vi "Process.vi"(4 "Normalize?":bool, 5 "Measurement Arrays IN":T1, 6 "Calibration Constant (1/deg)":dbl, 7 "Magnet position":dbl, 8 "Magnetic Field (mT)":dbl, 9 "Actual Measurement":T2={"Elapsed Time (s)"=0.0, "Hall sensor (mT)"=0.0, "LockIn A"=[1.33515e-05, 1.14442e-05, 1.90736e-05, 41.634], "LockIn B"=[1.33515e-05, 1.14442e-05, 1.90736e-05, 41.634], "Dc intensity (V)"=0.0, "Temperature (K)"=0.0}) -> (3 "Measurement Arrays OUT":T1)   [LabVIEW 2017]
uses:
  Meas_arrays.ctl
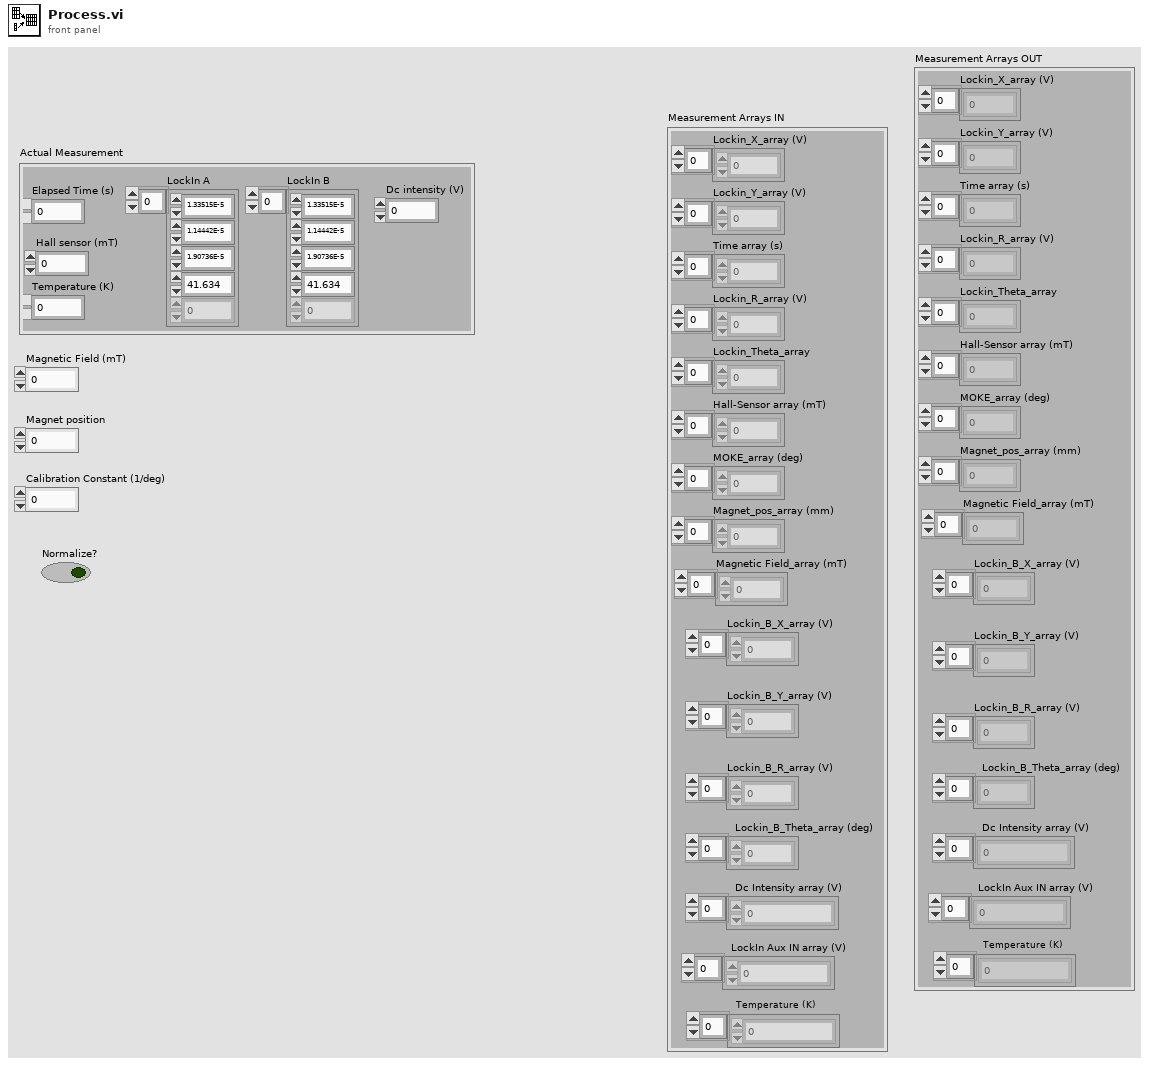
[diagram p1: front panel]
types:
  T1 = typedef "Meas_arrays.ctl" = cluster{"Lockin_X_array (V)":dbl[], "Lockin_Y_array (V)":dbl[], "Time array (s)":dbl[], "Lockin_R_array (V)":dbl[], "Lockin_Theta_array":dbl[], "Hall-Sensor array (mT)":dbl[], "MOKE_array (deg)":dbl[], "Magnet_pos_array (mm)":dbl[], "Magnetic Field_array (mT)":dbl[], "Lockin_B_X_array (V)":dbl[], "Lockin_B_Y_array (V)":dbl[], "Lockin_B_R_array (V)":dbl[], "Lockin_B_Theta_array (deg)":dbl[], "Dc Intensity array (V)":dbl[], "LockIn Aux IN array (V)":dbl[], "Temperature (K)":dbl[]}
  T2 = cluster{"Elapsed Time (s)":dbl, "Hall sensor (mT)":dbl, "LockIn A":dbl[], "LockIn B":dbl[], "Dc intensity (V)":dbl, "Temperature (K)":dbl}
  T3 = cluster{"Lockin_X_array (V)":dbl[], "Lockin_Y_array (V)":dbl[], "Time array (s)":dbl[], "Lockin_R_array (V)":dbl[], "Lockin_Theta_array":dbl[], "Hall-Sensor array (mT)":dbl[], "MOKE_array (deg)":dbl[], "Magnet_pos_array (mm)":dbl[], "Magnetic Field_array (mT)":dbl[], "Lockin_B_X_array (V)":dbl[], "Lockin_B_Y_array (V)":dbl[], "Lockin_B_R_array (V)":dbl[], "Lockin_B_Theta_array (deg)":dbl[], "Dc Intensity array (V)":dbl[], "LockIn Aux IN array (V)":dbl[], "Temperature (K)":dbl[]}
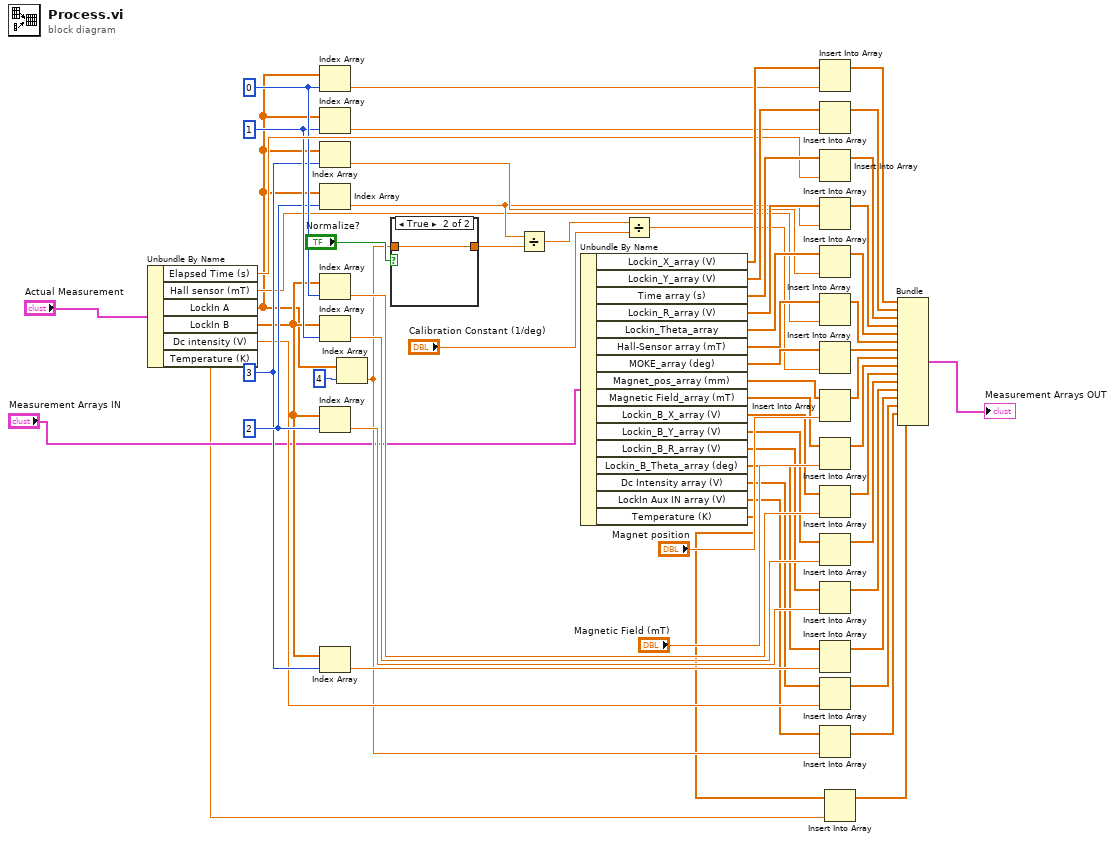
[diagram p0: block diagram]
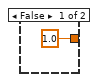
[diagram p2: hidden frame]
diagram:
  w32 = 3 ("index")
  w33 = 2 ("index")
  w34 = 1 ("index")
  w35 = 0 ("index")
  n1 = Unbundle By Name("Actual Measurement") -> ("Elapsed Time (s)"=w37:dbl, "Hall sensor (mT)"=w15:dbl, "LockIn A"=w11:dbl[], "LockIn B"=w31:dbl[], "Dc intensity (V)"=w14:dbl, "Temperature (K)"=w1:dbl)
  n2 = Index Array(array=w11, index=w35) -> (element=w39:dbl)
  n3 = Index Array(array=w11, index=w34) -> (element=w38:dbl)
  n4 = Index Array(array=w11, index=w32) -> (element=w36:dbl)
  n5 = Index Array(array=w11, index=w33) -> (element=w19:dbl)
  n6 = Index Array(array=w31, index=w35) -> (element=w30:dbl)
  n7 = Index Array(array=w31, index=w34) -> (element=w29:dbl)
  n8 = Index Array(array=w31, index=w33) -> (element=w28:dbl)
  n9 = Index Array(array=w31, index=w32) -> (element=w27:dbl)
  n10 = Index Array(array=w11, index=4) -> (element=w8:dbl)
  n11 = case shown="True" "Normalize?" {
    tunnel: [1.0 ("Dc intensity (V)") w64] -> w13
    tunnel: w8 -> [_ w64]
    frame False {
    }
    frame True {
    }
  }
  n12 = Divide(x=w19, y=w13) -> (x/y=w45:dbl)
  n13 = Unbundle By Name("Measurement Arrays IN") -> ("Lockin_X_array (V)"=w48:dbl[], "Lockin_Y_array (V)"=w49:dbl[], "Time array (s)"=w50:dbl[], "Lockin_R_array (V)"=w51:dbl[], "Lockin_Theta_array"=w52:dbl[], "Hall-Sensor array (mT)"=w53:dbl[], "MOKE_array (deg)"=w54:dbl[], "Magnet_pos_array (mm)"=w55:dbl[], "Magnetic Field_array (mT)"=w40:dbl[], "Lockin_B_X_array (V)"=w26:dbl[], "Lockin_B_Y_array (V)"=w25:dbl[], "Lockin_B_R_array (V)"=w24:dbl[], "Lockin_B_Theta_array (deg)"=w23:dbl[], "Dc Intensity array (V)"=w17:dbl[], "LockIn Aux IN array (V)"=w9:dbl[], "Temperature (K)"=w3:dbl[])
  n14 = Divide(x=w45, y="Calibration Constant (1/deg)") -> (x/y=w47:dbl)
  n15 = Insert Into Array(array=w48, new element=w39) -> (w57:dbl[])  [unwired: 1 in]
  n16 = Insert Into Array(array=w49, new element=w38) -> (w58:dbl[])  [unwired: 1 in]
  n17 = Insert Into Array(array=w50, new element=w37) -> (w56:dbl[])  [unwired: 1 in]
  n18 = Insert Into Array(array=w51, new element=w19) -> (w59:dbl[])  [unwired: 1 in]
  n19 = Insert Into Array(array=w52, new element=w36) -> (w60:dbl[])  [unwired: 1 in]
  n20 = Insert Into Array(array=w53, new element=w15) -> (w61:dbl[])  [unwired: 1 in]
  n21 = Insert Into Array(array=w54, new element=w47) -> (w62:dbl[])  [unwired: 1 in]
  n22 = Insert Into Array(array=w55, new element="Magnet position") -> (w43:dbl[])  [unwired: 1 in]
  n23 = Insert Into Array(array=w40, new element="Magnetic Field (mT)") -> (w41:dbl[])  [unwired: 1 in]
  n24 = Insert Into Array(array=w26, new element=w30) -> (w22:dbl[])  [unwired: 1 in]
  n25 = Insert Into Array(array=w25, new element=w29) -> (w21:dbl[])  [unwired: 1 in]
  n26 = Insert Into Array(array=w24, new element=w28) -> (w20:dbl[])  [unwired: 1 in]
  n27 = Insert Into Array(array=w23, new element=w27) -> (w18:dbl[])  [unwired: 1 in]
  n28 = Insert Into Array(array=w17, new element=w14) -> (w16:dbl[])  [unwired: 1 in]
  n29 = Insert Into Array(array=w9, new element=w8) -> (w7:dbl[])  [unwired: 1 in]
  n30 = Insert Into Array(array=w3, new element=w1) -> (w2:dbl[])  [unwired: 1 in]
  n31 = Bundle("Lockin_X_array (V)"=w57, "Lockin_Y_array (V)"=w58, "Time array (s)"=w56, "Lockin_R_array (V)"=w59, "Lockin_Theta_array"=w60, "Hall-Sensor array (mT)"=w61, "MOKE_array (deg)"=w62, "Magnet_pos_array (mm)"=w43, "Magnetic Field_array (mT)"=w41, "Lockin_B_X_array (V)"=w22, "Lockin_B_Y_array (V)"=w21, "Lockin_B_R_array (V)"=w20, "Lockin_B_Theta_array (deg)"=w18, "Dc Intensity array (V)"=w16, "LockIn Aux IN array (V)"=w7, "Temperature (K)"=w2) -> (→"Measurement Arrays OUT":T3)  [unwired: 1 in]
